vi "get Period.vi"(3 "Metronome Actor in":refnum<class "Metronome Actor.lvclass">) -> (0 "Period [ms]":i32)   [LabVIEW 2015, in "Metronome Actor.lvclass"]
uses:
  Metronome Actor.lvclass
  Metronome Actor.lvclass/Metronome Actor.ctl
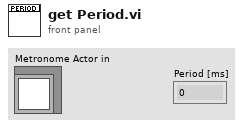
[diagram p1: front panel]
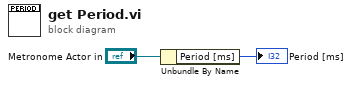
[diagram p0: block diagram]
diagram:
  n1 = Unbundle By Name("Metronome Actor in") -> ("Period [ms]"=→"Period [ms]":i32)
